vi "Spill alarm change.vi"(8 "error in":errorcluster, 9 "Model Data before update":T1, 10 "Model Data after update":T1) -> (0 "error out":errorcluster, 1 "Model Data after update out":T1, 2 "Spill alarm value change":bool, 3 "Spill alarm turned on":bool)   [LabVIEW 2015, in "Model.lvlib"]
uses:
  Model.lvlib
  TypeDefs/Model Data.ctl
  TypeDefs/PL Settings.ctl
  TypeDefs/PL UI Refs.ctl
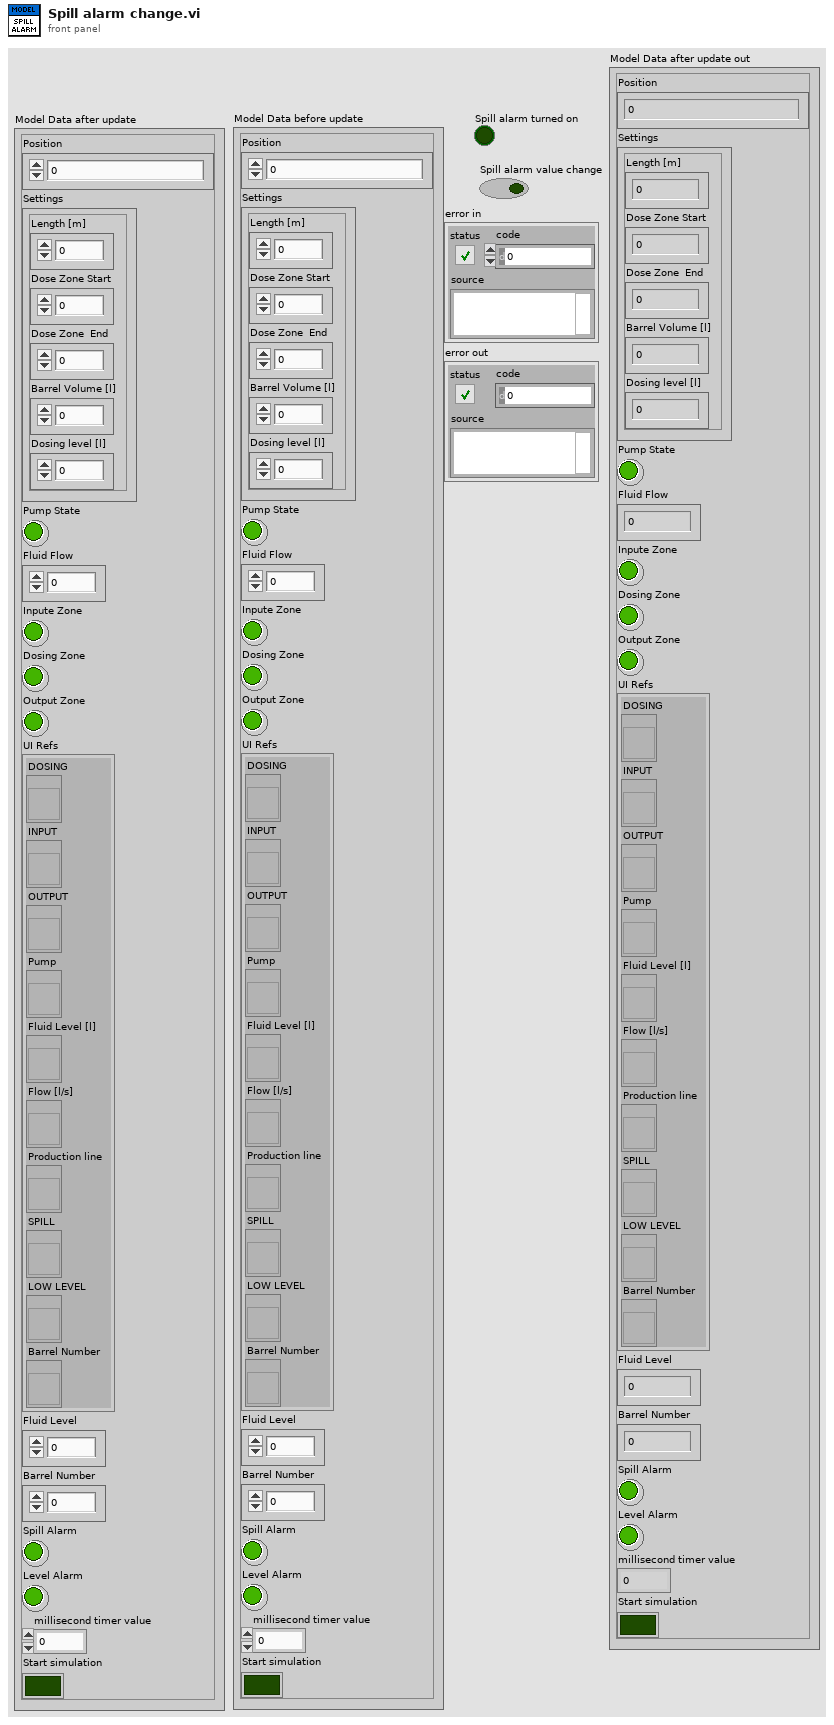
[diagram p1: front panel]
types:
  T1 = typedef "Model.lvlib/Model Data.ctl" = cluster{"Position":dbl, "Settings":T2, "Pump State":bool, "Fluid Flow":dbl, "Inpute Zone":bool, "Dosing Zone":bool, "Output Zone":bool, "UI Refs":T3, "Fluid Level":dbl, "Barrel Number":i32, "Spill Alarm":bool, "Level Alarm":bool, "millisecond timer value":u32, "Start simulation":bool}
  T2 = typedef "Model.lvlib/PL Settings.ctl" = cluster{"Length [m]":dbl, "Dose Zone Start":dbl, "Dose Zone  End":dbl, "Barrel Volume [l]":dbl, "Dosing level [l]":dbl}
  T3 = typedef "Model.lvlib/PL UI Refs.ctl" = cluster{"DOSING":refnum<vi>, "INPUT":refnum<vi>, "OUTPUT":refnum<vi>, "Pump":refnum<vi>, "Fluid Level [l]":refnum<vi>, "Flow [l/s]":refnum<vi>, "Production line":refnum<vi>, "SPILL":refnum<vi>, "LOW LEVEL":refnum<vi>, "Barrel Number":refnum<vi>}
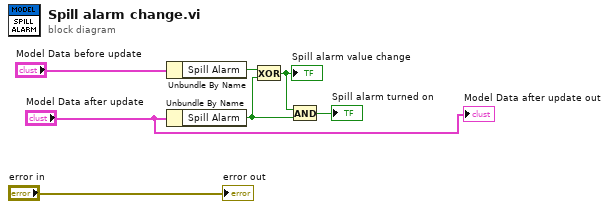
[diagram p0: block diagram]
diagram:
  n1 = Unbundle By Name("Model Data before update") -> ("Spill Alarm"=w4:bool)
  n2 = Unbundle By Name("Model Data after update") -> ("Spill Alarm"=w6:bool)
  n3 = Exclusive Or(1:w6, 2:w4) -> (0:w5:bool)
  "Spill alarm value change" <- w5
  n4 = And(x=w5, y=w6) -> (x .and. y?=→"Spill alarm turned on":bool)
  "error out" <- "error in"
  "Model Data after update out" <- "Model Data after update"
